vi "read timing source name.vi"(8 "error in":errorcluster, 11 "module in":refnum<class "asynchronous execution module runtime.lvclass">) -> (0 "error out":errorcluster, 2 "timing source":refnum<class "TBM timing source.lvclass">, 3 "module out":refnum<class "asynchronous execution module runtime.lvclass">)   [LabVIEW 2013, in "asynchronous execution module runtime.lvclass"]
uses:
  asynchronous execution module runtime.lvclass
  <vilib>/NI/Module Timing Source/timing source/TBM timing source.lvclass
  asynchronous execution module runtime.lvclass/asynchronous execution module runtime.ctl
  <vilib>/NI/Tag Bus Module Framework/runtime/TBM module execution interface.lvclass
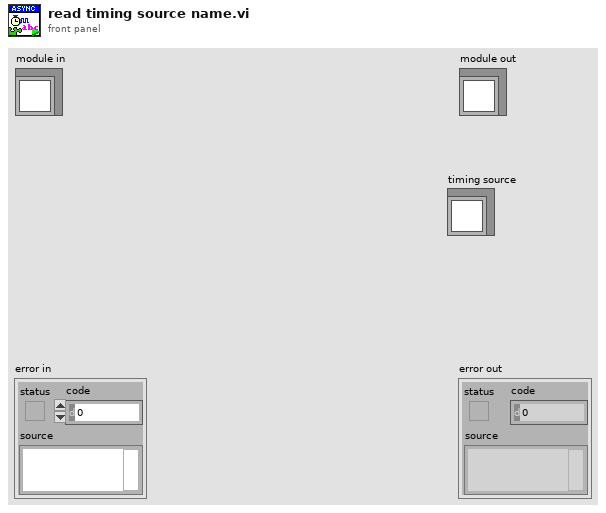
[diagram p1: front panel]
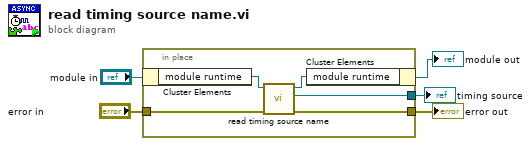
[diagram p0: block diagram]
diagram:
  n1 = in-place {
    in-place-border: "error in" -> [w10]
    in-place-border: [w9] -> w4
    in-place-border: [w8] -> w1
    n2 = in-place-cluster #1("module in") -> ("module runtime"=w6:refnum<class "TBM module execution interface.lvclass">)
    n3 = call-dynamic "read timing source name.vi"("error in"=w10, "module in"=w6) -> ("error out"=w9:errorcluster, "timing source"=w8:refnum<class "TBM timing source.lvclass">, "module out"=w7:refnum<class "TBM module execution interface.lvclass">)  [unwired: 7 in]
    n4 = in-place-cluster #1("module runtime"=w7) -> (→"module out":refnum<class "asynchronous execution module runtime.lvclass">)
  }
  "error out" <- w4
  "timing source" <- w1
